vi "_Add Array of JSON Objects to JSON.vi"(6 "Pretty Print?":bool, 7 "JSON Object Name":string, 8 "error in (no error)":errorcluster, 9 "JSON Array Name":string, 10 "JSON Objects":string[](array[string]), 11 "JSON":string) -> (0 "error out":errorcluster, 3 "<JSON>":string)   [LabVIEW 2021]
uses:
  <vilib>/JDP Science/JSONtext/support/Format JSON Array Text.vi
  <vilib>/JDP Science/JSONtext/support/Format JSON Object.vi
  <vilib>/JDP Science/JSONtext/Get all Object Items.vi
  <vilib>/JDP Science/JSONtext/Set Multiple Object Items.vi
  <vilib>/JDP Science/JSONtext/JSONtext.lvlib
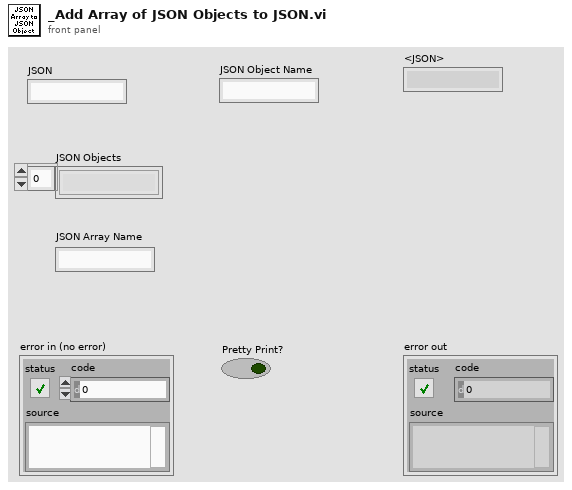
[diagram p1: front panel]
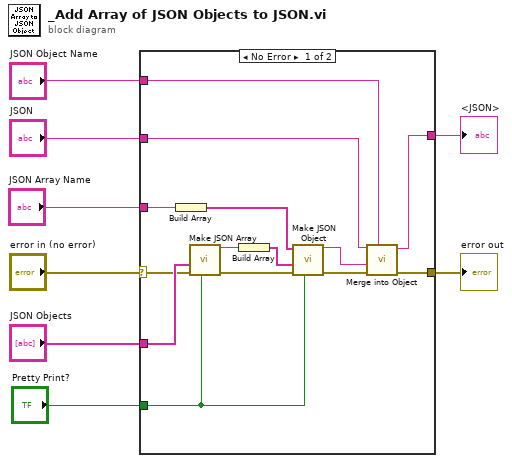
[diagram p0: block diagram]
diagram:
  n1 = case shown="No Error" "error in (no error)" {
    selector: "error in (no error)" -> [w11 w23]
    tunnel: "Pretty Print?" -> [w22 _]
    tunnel: "JSON Object Name" -> [w21 _]
    tunnel: "JSON" -> [w20 w24]
    tunnel: [w14 w23] -> w5
    tunnel: [w13 w24] -> w4
    tunnel: "JSON Objects" -> [w12 _]
    tunnel: "JSON Array Name" -> [w10 _]
    frame No Error {
      n2 = Build Array(w10) -> (w9:string[])
      n3 = call <vilib>:"Make JSON Array.vi"("Pretty Print?"=w22, "error in (no error)"=w11, "JSON Elements"=w12) -> ("error out"=w15:errorcluster, "<JSON>"=w19:string)  [unwired: 7 in]
      n4 = Build Array(w19) -> (w18:string[])
      n5 = call <vilib>:"Make JSON Object.vi"("Pretty Print?"=w22, "error in (no error)"=w15, "JSON Items"=w18, "Item Names"=w9) -> ("error out"=w17:errorcluster, "<JSON>"=w16:string)  [unwired: 6 in]
      n6 = call <vilib>:"Merge into Object.vi"("$Path or Item Name"=w21, "error in (no error)"=w17, "JSON Object to Merge"=w16, "JSON"=w20) -> ("error out"=w14:errorcluster, "<JSON>"=w13:string)  [unwired: 5 in]
    }
    frame Error {
    }
  }
  "error out" <- w5
  "<JSON>" <- w4
